vi "G4SubTemplate_Simple_5x6x5_ReadProperty.vi"(0 "reference in":refnum<class "G4SubTemplate_Simple_5x6x5.lvclass">, 11 "Error In":errorcluster) -> (4 "reference out":refnum<class "G4SubTemplate_Simple_5x6x5.lvclass">, 8 "Property":dbl, 15 "Error Out":errorcluster)   [LabVIEW 2020]
uses:
  <resource>/Framework/Providers/Open_GDS/ClassProviders/Provider_EndevoGOOP400/Templates/G4SubTemplate_Simple_5x6x5/G4SubTemplate_Simple_5x6x5.lvclass
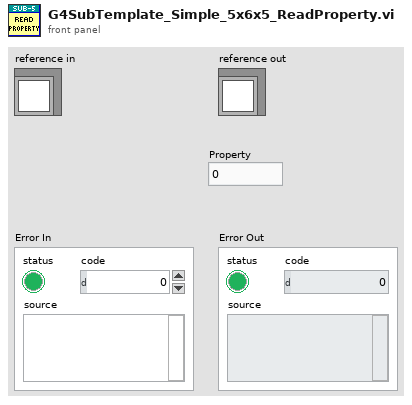
[diagram p1: front panel]
types:
  T1 = typedef "G4SubTemplate_Simple_5x6x5.lvclass/ObjectAttributes.ctl" = cluster{"Attribute1":dbl}
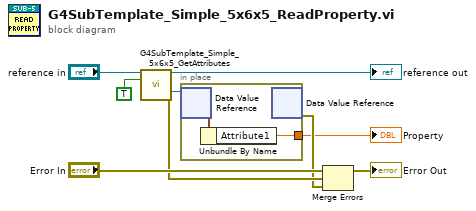
[diagram p0: block diagram]
diagram:
  n1 = call <resource>:"G4SubTemplate_Simple_5x6x5_GetAttributes.vi"("reference in"="reference in", "OnlyGetDvrReference(False)"=TRUE) -> ("reference out"=→"reference out":refnum<class "G4SubTemplate_Simple_5x6x5.lvclass">, "DataRef"=w2:refnum<data-value>, "Error Out"=w8:errorcluster)  [unwired: 10 in, 1 out]
  n2 = in-place {
    in-place-border: [w11] -> w1
    n3 = in-place-dvr #1(w2) -> (w10:T1)  [unwired: 1 out]
    n4 = Unbundle By Name(w10) -> ("Attribute1"=w11:dbl)
    n5 = in-place-dvr #1() -> (w6:errorcluster)  [unwired: 1 in, 1 out]
  }
  "Property" <- w1
  n6 = Merge Errors("Error In", w8, w6) -> (→"Error Out":errorcluster)
